vi "Process EH Error.vi"(8 "error in (no error)":errorcluster, 10 "Error to process":errorcluster, 11 "Ancestor in":refnum<class "Ancestor.lvclass">) -> (0 "error out":errorcluster, 3 "Ancestor out":refnum<class "Ancestor.lvclass">)   [LabVIEW 2026, in "TALOS.lvlib" / "Ancestor.lvlib" / "Ancestor.lvclass"]
uses:
  Ancestor.lvclass
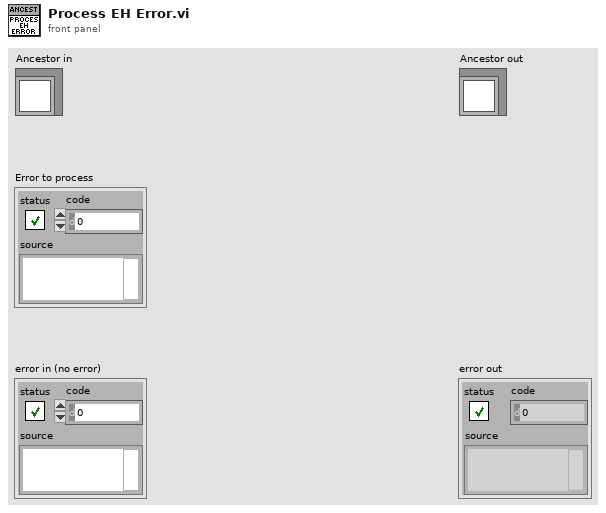
[diagram p1: front panel]
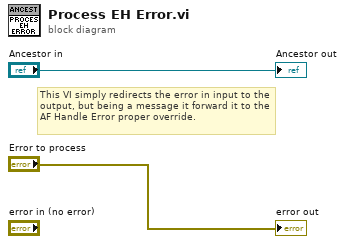
[diagram p0: block diagram]
diagram:
  # "This VI simply redirects the error in input to the output, but being a message it forward it to the AF Handle Error proper override."
  "error out" <- "Error to process"
  "Ancestor out" <- "Ancestor in"
